vi "Valid Guesses--constant.vi"() -> (2 "Valid Guesses (array)":string[](array[string]), 3 "Valid Guesses (set)":set{string}(c389))   [LabVIEW 2022 SP3, in "Wordle Engine.lvlib"]
doc: "All valid guesses for the Wordle word. The target word was selected from an undisclosed subset of the words in this list.\n\nNote that this VI returns the list as both an array of strings, and a set of strings."
uses:
  Wordle Engine.lvlib
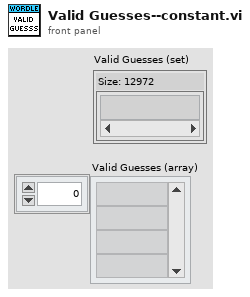
[diagram p1: front panel]
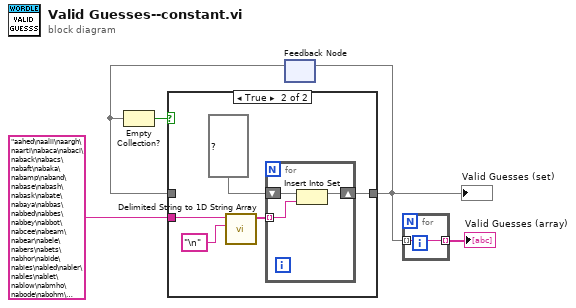
[diagram p0: block diagram]
diagram:
  n1 = feedback #1() -> (w3:set{string})  [unwired: 1 in]
  n2 = Empty Collection?(1:w3) -> (0:w5:bool)
  n3 = case shown="True" w5 {
    tunnel: "aahed\naalii\naargh\naarti\nabaca\nabaci\naback\nabacs\nabaft\nabaka\nabamp\naband\nabase\nabash\nabask\nabate\nabaya\nabbas\nabbed\nabbes\nabbey\nabbot\nabcee\nabeam\nabear\nabele\nabers\nabets\nabhor\nabide\nabies\nabled\nabler\nables\nablet\nablow\nabmho\nabode\nabohm\naboil\naboma\naboon\nabord\nabore\nabort\nabout\nabove\nabram\nabray\nabrim\nabrin\nabris\nabsey\nabsit\nabuna\nabune\nabuse\nabuts\nabuzz\nabyes\nabysm\nabyss\nacais\nacari\naccas\naccoy\nacerb\nacers\naceta\nachar\nached\naches\nachoo\nacids\nacidy\nacing\nacini\nackee\nacker\nacmes\nacmic\nacned\nacnes\nacock\nacold\nacorn\nacred\nacres\nacrid\nacros\nacted\nactin\nacton\nactor\nacute\nacyls\nadage\nadapt\nadaws\nadays\n..." -> [_ w11]
    tunnel: [w6 w8] -> w2
    tunnel: w3 -> [w6 _]
    frame False {
    }
    frame True {
      n4 = call <vilib>:"Delimited String to 1D String Array.vi"("delimiter"="\n", "delimited string"=w11) -> ("string array"=w10:string[])  [unwired: 9 in]
      n5 = for {
        tunnel: w10 -> [w12] mode=indexing
        shift-right: [w14] -> w8
        shift-left: set{string} {} ("Valid Guesses") -> [w13]
        n6 = Insert Into Set(10:w12, 11:w13) -> (3:w14:set{string})  [unwired: 1 out]
      }
    }
  }
  "Valid Guesses (set)" <- w2
  n7 = feedback-in #1(w2) -> ()
  n8 = for {
    tunnel: [w15] -> w1 mode=indexing
    tunnel: w2 -> [w15] mode=indexing
  }
  "Valid Guesses (array)" <- w1
